vi "Initiate assembly.vi"(0 "Database Entry in":refnum<class "Database Entry.lvclass">, 11 "error in (no error)":errorcluster) -> (2 "Feet check":bool, 4 "Database Entry out":refnum<class "Database Entry.lvclass">, 6 "Module?":bool, 8 "Abort out":bool, 15 "error out":errorcluster)   [LabVIEW 2021, in "Database Entry.lvclass"]
uses:
  Database Entry.lvclass
  Database Entry.lvclass/Database Entry.ctl
  <vilib>/Utility/file.llb/Read Delimited Spreadsheet (string).vi
  <vilib>/JDP Science/JDP Science Common Utilities/JDP Utility.lvlib
panel:
  out "Now assembling...":string
  in  "Abort":bool
  in  "Relative humidity":string
  in  "Temperature (C)":string
  in  "ROC version":u16(ring)=1 items=["HGCROCV3b-2", "HGCROCV3b-4", "HGCROCV3c", "Preseries"]
  in  "Adhesive":u16(ring) items=["Hybrid", "Transfer tape only", "Epoxy only"]
  in  "Module Type":u16(ring) items=["CMU,LD,Full,200,CuW", "CMU,LD,Full,300,CuW", "CMU,LD,Full,200,Ti", "CMU,LD,Full,300,Ti", "CMU,LD,Full,200,CF", "CMU,LD,Full,300,CF"]
  in  "Operator":u16(ring) items=["jestein", "JonasRoemer", "simurthy", "cmumac"]
  out "Status":dbl[][](array[numeric])
  in  "Assembly Region":cluster{"1":bool, "2":bool, "3":bool, "4":bool}
  in  "Submit":bool
  # "(To update existing modules, click 'Submit' without any selection and skipt to the Manual Assembly DB.)"
  # "Tray Slot 1"
  # "Tray Slot 2"
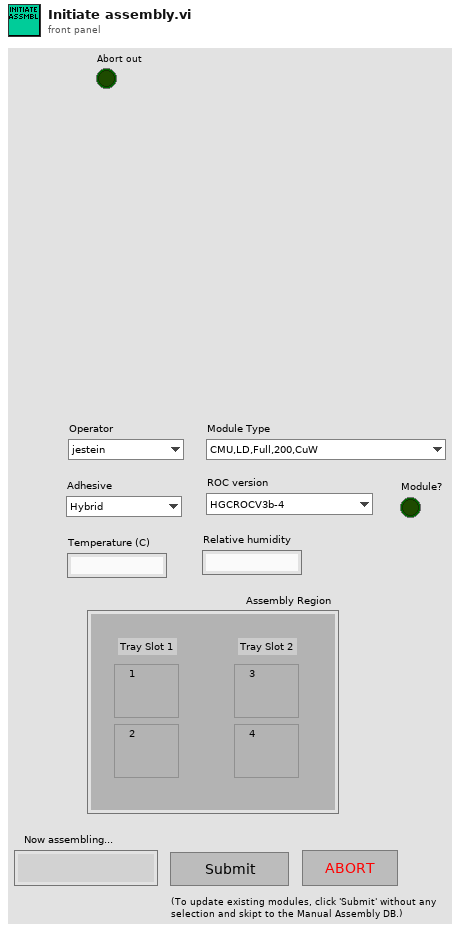
[diagram p1: front panel]
types:
  T1 = typedef "File Paths.ctl" = cluster{"Glue Pattern Folder":path, "Carrier Tray Folder":path, "Pick Up Tool Fixture Folder":path, "Components Folder":path, "Bellows Tool Offset.txt":path, "Pick Up Tool Offset.txt":path, "Dispense Tip Offset.txt":path, "Log Files":path, "Gantry Assembly Map.txt":path, "Syringe and offset map.txt":path, "Controllers Folder":path, "Local dbase config":path}
  T2 = cluster{"Temperature (C)":string, "Relative humidity":string}
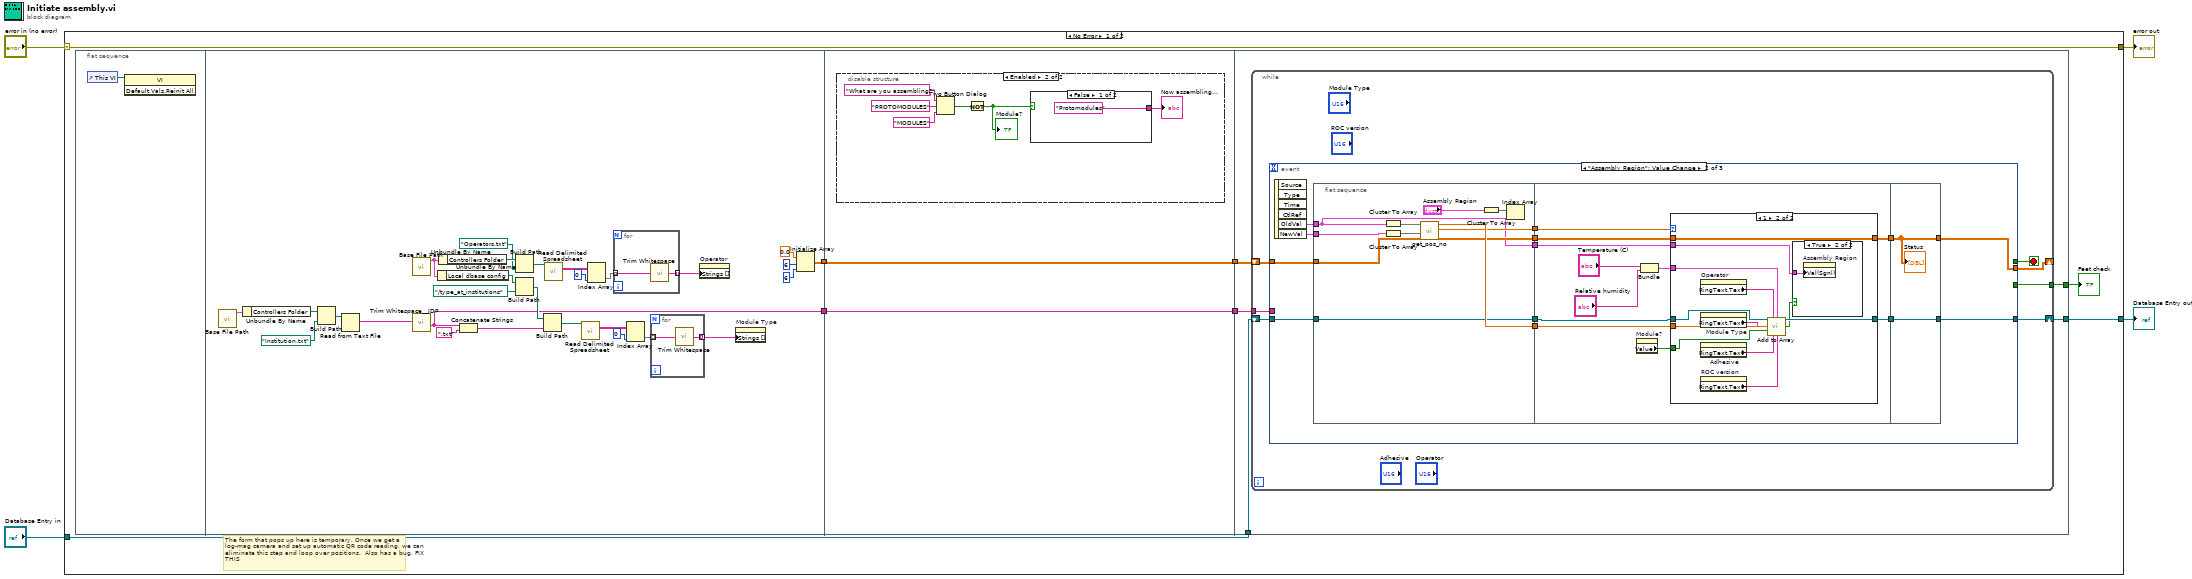
[diagram p0: block diagram]
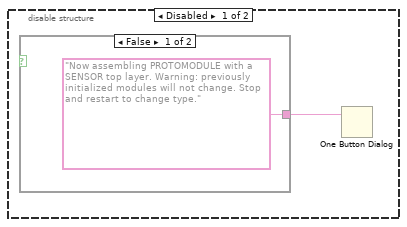
[diagram p2: hidden frame]
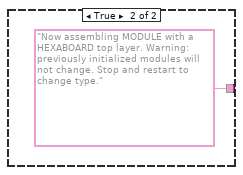
[diagram p3: hidden frame]
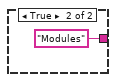
[diagram p4: hidden frame]
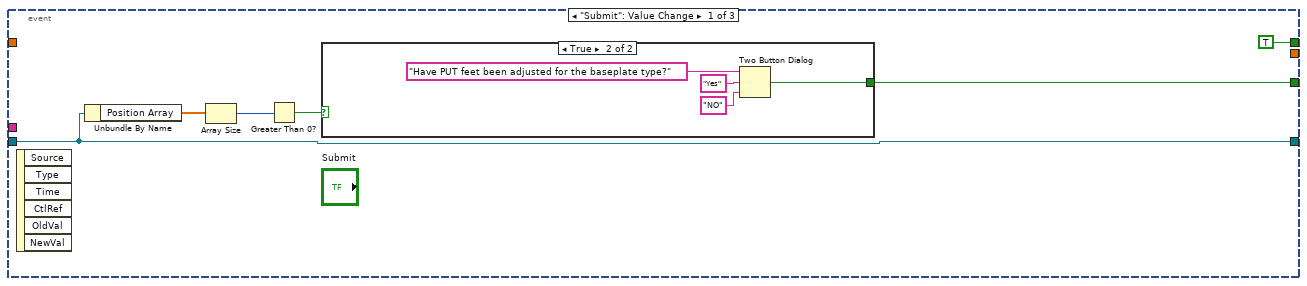
[diagram p5: hidden frame]
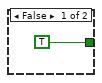
[diagram p6: hidden frame]
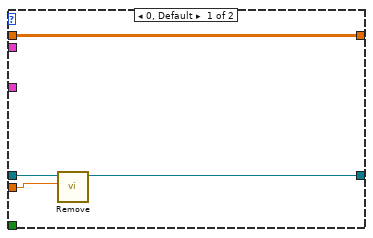
[diagram p7: hidden frame]
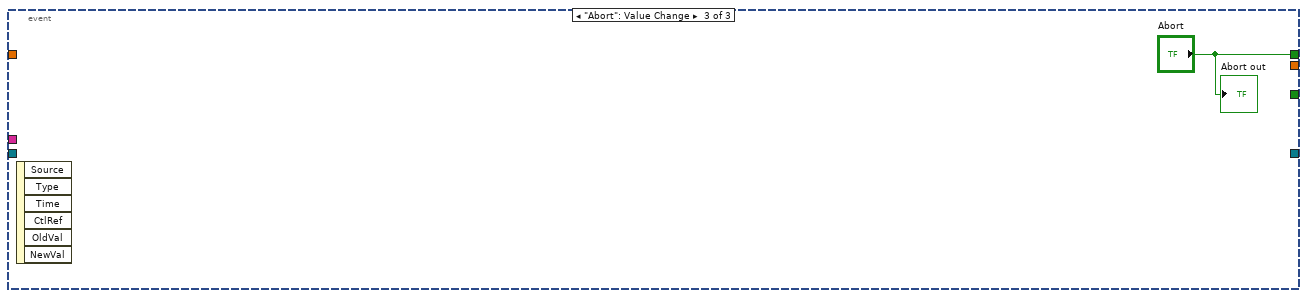
[diagram p9: hidden frame]
diagram:
  n1 = case shown="No Error" "error in (no error)" {
    selector: "error in (no error)" -> [w5 w138]
    tunnel: [w5 w138] -> w3
    tunnel: [w6 w137] -> w1
    tunnel: "Database Entry in" -> [w12 w137]
    frame No Error {
      # "The form that pops up here is temporary. Once we get a log-mag camera and set up automatic QR code reading, we can eliminate this step and loop over positions.  Also has a bug. FIX THIS"
      n2 = flat-sequence {
        tunnel: [w32] -> w10
        tunnel: [w21] -> w8
        tunnel: w10 -> [w47]
        tunnel: [w47] -> w9
        tunnel: w8 -> [w46]
        tunnel: [w46] -> w7
        tunnel: w9 -> [w62]
        tunnel: w7 -> [w61]
        tunnel: w12 -> [w63]
        tunnel: [w60] -> w6
        tunnel: [w59] -> w11
        frame #0 {
          n3 = control-ref of="This VI"() -> (w13:refnum<vi>)
          n4 = invoke class="VI" method="Default Vals.Reinit All"(reference=w13) -> ()  [unwired: 2 in, 3 out]
        }
        frame #1 {
          n5 = call "Base File Path.vi"() -> ("Paths Out"=w41:T1)  [unwired: 11 in]
          n6 = Unbundle By Name(w41) -> ("Controllers Folder"=w23:path)
          n7 = Build Path(base path=w23, name or relative path=path "Institution.txt") -> (appended path=w39:path)
          n8 = Read from Text File(file (use dialog)=w39) -> (text=w38:string)  [unwired: 3 in, 3 out]
          n9 = call "Base File Path.vi"() -> ("Paths Out"=w28:T1)  [unwired: 11 in]
          n10 = call <vilib>:"Trim Whitespace__JDP.vi"("String in"=w38) -> ("String out"=w21:string)  [unwired: 6 in]
          n11 = Unbundle By Name(w28) -> ("Local dbase config"=w27:path)
          n12 = Unbundle By Name(w28) -> ("Controllers Folder"=w37:path)
          n13 = Concatenate Strings(w21, ".txt" ("string")) -> (w19:string)
          n14 = Build Path(base path=w37, name or relative path=path "Operators.txt") -> (appended path=w35:path)
          n15 = Build Path(base path=w27, name or relative path=path "../type_at_institutions") -> (appended path=w24:path)
          n16 = Build Path(base path=w24, name or relative path=w19) -> (appended path=w22:path)
          n17 = call-poly <vilib>:"Read Delimited Spreadsheet.vi"("file path (dialog if empty)"=w35) -> ("all rows"=w34:string[][])  [unwired: 9 in, 5 out]
          n18 = call-poly <vilib>:"Read Delimited Spreadsheet.vi"("file path (dialog if empty)"=w22) -> ("all rows"=w18:string[][])  [unwired: 9 in, 5 out]
          n19 = Index Array(array=w34, index (col)=0 ("disabled index (col)")) -> (element=w17:string[])  [unwired: 1 in]
          n20 = for {
            tunnel: w17 -> [w45] mode=indexing
            tunnel: [w44] -> w16 mode=indexing
            n21 = call <vilib>:"Trim Whitespace.vi"("string"=w45) -> ("trimmed string"=w44:string)  [unwired: 1 in]
          }
          n22 = Index Array(array=w18, index (col)=0 ("disabled index (col)")) -> (element=w15:string[])  [unwired: 1 in]
          n23 = for {
            tunnel: w15 -> [w43] mode=indexing
            tunnel: [w42] -> w14 mode=indexing
            n24 = call <vilib>:"Trim Whitespace.vi"("string"=w43) -> ("trimmed string"=w42:string)  [unwired: 1 in]
          }
          n25 = property on="Operator" class="Ring (strict)"("Strings []"=w16) -> ()  [unwired: 2 in, 2 out]
          n26 = property on="Module Type" class="Ring (strict)"("Strings []"=w14) -> ()  [unwired: 2 in, 2 out]
          n27 = Initialize Array(0.0 ("element"), 6 ("dimension size"), 6 ("dimension size")) -> (w32:dbl[][])
        }
        frame #2 {
          n28 = disable-structure shown="Enabled" {
            frame Disabled {
              n29 = case shown="False" {
                selector: _ -> [_ _]
                tunnel: ["Now assembling PROTOMODULE with a SENSOR top layer. Warning: previously initialized modules will not change. Stop and restart to change type." "Now assembling MODULE with a HEXABOARD top layer. Warning: previously initialized modules will not change. Stop and restart to change type."] -> w48
                frame False {
                }
                frame True {
                }
              }
              n30 = One Button Dialog(message=w48) -> ()  [unwired: 1 in, 1 out]
            }
            frame Enabled {
              n31 = Two Button Dialog(message="What are you assembling?", 1:"MODULES" ("F button name (\"Cancel\")"), 2:"PROTOMODULES" ("T button name (\"OK\")")) -> (T button?=w53:bool)
              n32 = Not(x=w53) -> (.not. x?=w52:bool)
              "Module?" <- w52
              n33 = case shown="False" w52 {
                tunnel: ["Protomodules" ("Now assembling...") "Modules" ("Now assembling...")] -> w51
                frame False {
                }
                frame True {
                }
              }
              "Now assembling..." <- w51
            }
          }
        }
        frame #3 {
          n34 = while {
            shift-right: [w70] -> w60
            shift-left: w63 -> [w67]
            shift-right: [w68] -> _
            shift-left: w62 -> [w69]
            tunnel: w61 -> [w66]
            tunnel: [w64] -> w59
            stop <- w65 stop-if-true
            n35 = event shown="[1] \"Assembly Region\": Value Change" {
              selector: _ -> [_ _ _]
              dyn-events: _ -> [_ _ _]
              timeout: _ -> [_ _ _]
              tunnel: [TRUE ("T button?") _ "Abort"] -> w65
              tunnel: w67 -> [w74 w88 _]
              tunnel: [w74 w85 _] -> w70
              tunnel: w69 -> [_ w93 _]
              tunnel: [_ w89 _] -> w68
              tunnel: w66 -> [_ _ _]
              tunnel: [w75 _ _] -> w64
              event "Submit": Value Change {
                n36 = event-data() -> ()  [unwired: 1 in, 6 out]
                n37 = Unbundle By Name(w74) -> ("Position Array"=w73:dbl[])
                n38 = Array Size(array=w73) -> (size(s)=w72:i32)
                n39 = Greater Than 0?(x=w72) -> (x > 0?=w71:bool)
                n40 = case shown="True" w71 {
                  tunnel: [TRUE ("T button?") w78] -> w75
                  frame False {
                  }
                  frame True {
                    n41 = Two Button Dialog(message="Have PUT feet been adjusted for the baseplate type?", 1:"NO" ("F button name (\"Cancel\")"), 2:"Yes" ("T button name (\"OK\")")) -> (T button?=w78:bool)
                  }
                }
              }
              event "Assembly Region": Value Change {
                n42 = event-data() -> ("OldVal"=w82:cluster{"1":bool, "2":bool, "3":bool, "4":bool}, "NewVal"=w94:cluster{"1":bool, "2":bool, "3":bool, "4":bool})  [unwired: 1 in, 4 out]
                n43 = flat-sequence {
                  tunnel: w94 -> [w104]
                  tunnel: w82 -> [w95]
                  tunnel: w93 -> [w100]
                  tunnel: [w97] -> w91
                  tunnel: [w99] -> w90
                  tunnel: w88 -> [w98]
                  tunnel: [w98] -> w87
                  tunnel: [w96] -> w86
                  tunnel: [w95] -> w83
                  tunnel: [w115] -> w92
                  tunnel: w91 -> [w116]
                  tunnel: w90 -> [w113]
                  tunnel: w87 -> [w114]
                  tunnel: w86 -> [w112]
                  tunnel: [w111] -> w84
                  tunnel: w83 -> [w110]
                  tunnel: w92 -> [w135]
                  tunnel: [w135] -> w89
                  tunnel: [w134] -> w85
                  tunnel: w84 -> [w134]
                  frame #0 {
                    n44 = Cluster To Array(cluster=w95) -> (array=w101:bool[])
                    n45 = Cluster To Array(cluster=w104) -> (array=w102:bool[])
                    n46 = call "get_pos_no.vi"("Status Old"=w100, "Array New Status"=w102, "Array Old Status"=w101) -> ("Status New"=w97:dbl[][], "State"=w96:dbl, "Position ID"=w99:dbl)  [unwired: 2 in]
                    n47 = Cluster To Array(cluster="Assembly Region") -> (array=w105:bool[])
                    n48 = Index Array(array=w105) -> ()  [unwired: 1 in, 1 out]
                  }
                  frame #1 {
                    n49 = property on="Module?" class="Bool (strict)"() -> ("Value"=w109:bool)  [unwired: 2 in, 2 out]
                    n50 = Bundle("Temperature (C)"="Temperature (C)", "Relative humidity"="Relative humidity") -> (w106:T2)  [unwired: 1 in]
                    n51 = case shown="1" w112 {
                      tunnel: w116 -> [w117 w132]
                      tunnel: [w117 w132] -> w115
                      tunnel: w114 -> [w120 w131]
                      tunnel: [w119 w130] -> w111
                      tunnel: w113 -> [w118 w129]
                      tunnel: w109 -> [_ w128]
                      tunnel: w110 -> [_ w122]
                      tunnel: w106 -> [_ w121]
                      frame 0, Default {
                        n52 = call "Remove.vi"("Index"=w118, "Database Entry in"=w120) -> ("Database Entry out"=w119:refnum<class "Database Entry.lvclass">)  [unwired: 8 in, 1 out]
                      }
                      frame 1 {
                        n53 = property on="Operator" class="Ring (strict)"() -> ("RingText.Text"=w127:string)  [unwired: 2 in, 2 out]
                        n54 = property on="Module Type" class="Ring (strict)"() -> ("RingText.Text"=w126:string)  [unwired: 2 in, 2 out]
                        n55 = property on="Adhesive" class="Ring (strict)"() -> ("RingText.Text"=w125:string)  [unwired: 2 in, 2 out]
                        n56 = property on="ROC version" class="Ring (strict)"() -> ("RingText.Text"=w124:string)  [unwired: 2 in, 2 out]
                        n57 = call "Add to Array.vi"("Database Entry in"=w131, "Operator"=w127, "Temp and RelHumidity"=w121, "Position Index"=w129, "Module type"=w126, "Module?"=w128, "Adhesive"=w125, "ROC version"=w124) -> ("Database Entry out"=w130:refnum<class "Database Entry.lvclass">, "Position cancelled?"=w123:bool)  [unwired: 5 in, 1 out]
                        n58 = case shown="True" w123 {
                          tunnel: w122 -> [_ w133]
                          frame False {
                          }
                          frame True {
                            n59 = property on="Assembly Region" class="Clust (strict)"("Val(Sgnl)"=w133) -> ()  [unwired: 2 in, 2 out]
                          }
                        }
                      }
                    }
                  }
                  frame #2 {
                    "Status" <- w135
                  }
                }
              }
              event "Abort": Value Change {
                n60 = event-data() -> ()  [unwired: 1 in, 6 out]
                "Abort out" <- "Abort"
              }
            }
          }
        }
      }
      "Feet check" <- w11
    }
    frame Error {
    }
  }
  "error out" <- w3
  "Database Entry out" <- w1
